vi "GET_Issues.vi"(6 "progress ref":refnum<vi>, 8 "error in (no error)":errorcluster, 11 "series_class in":refnum<class "series_class.lvclass">) -> (0 "error out":errorcluster, 3 "series_class out":refnum<class "series_class.lvclass">)   [LabVIEW 2024, in "series_class.lvclass"]
uses:
  series_class.lvclass
  series_class.lvclass/series_class.ctl
  issue_class/issue_class.lvclass
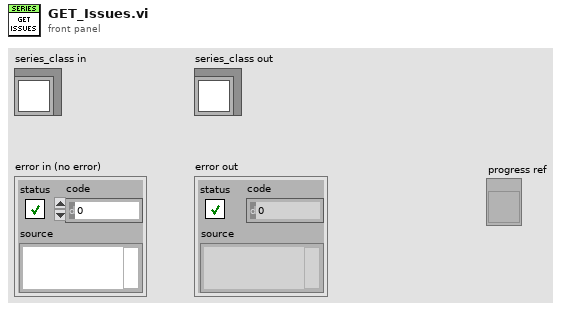
[diagram p1: front panel]
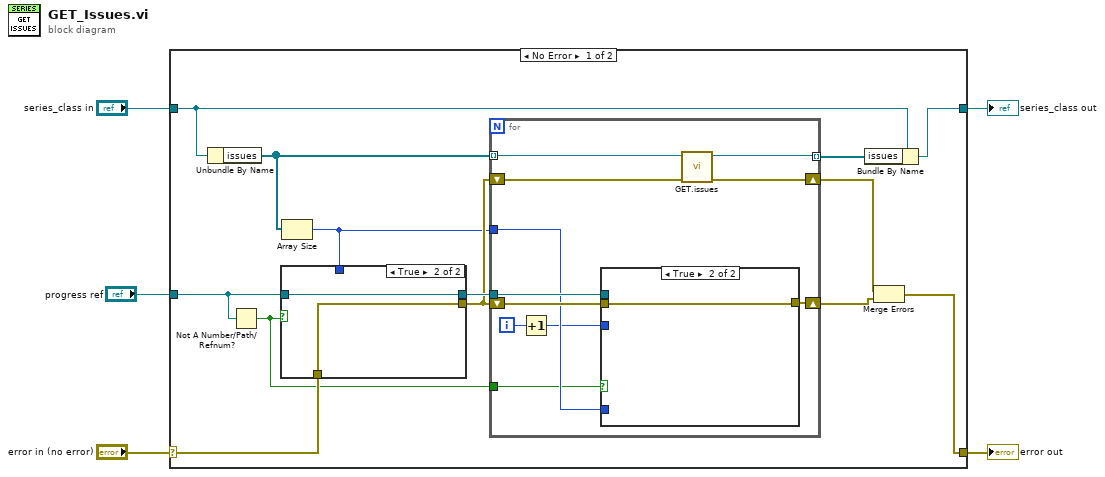
[diagram p0: block diagram]
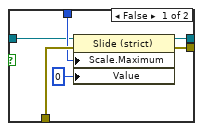
[diagram p2: hidden frame]
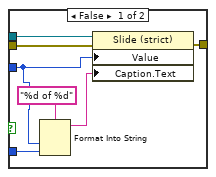
[diagram p3: hidden frame]
diagram:
  n1 = case shown="No Error" "error in (no error)" {
    selector: "error in (no error)" -> [w13 w47]
    tunnel: [w9 w47] -> w4
    tunnel: [w17 w46] -> w2
    tunnel: "series_class in" -> [w18 w46]
    tunnel: "progress ref" -> [w7 _]
    frame No Error {
      n2 = Unbundle By Name(w18) -> ("issues"=w14:refnum<class "issue_class.lvclass">[])
      n3 = Not A Number/Path/Refnum?(number/path/refnum=w7) -> (NaN/Path/Refnum?=w6:bool)
      n4 = Array Size(array=w14) -> (size(s)=w8:i32)
      n5 = case shown="True" w6 {
        tunnel: [w23 w26] -> w15
        tunnel: w13 -> [w22 w25]
        tunnel: [w21 w25] -> w12
        tunnel: w8 -> [w20 _]
        tunnel: w7 -> [w19 w26]
        frame False {
          n6 = property class="Slide (strict)"(reference=w19, error in=w22, "Scale.Maximum"=w20, "Value"=0) -> (reference out=w23:refnum<vi>, error out=w21:errorcluster)
        }
        frame True {
        }
      }
      n7 = for {
        tunnel: w14 -> [w37] mode=indexing
        tunnel: [w36] -> w16 mode=indexing
        shift-right: [w34] -> w11
        shift-left: w12 -> [w35]
        tunnel: w15 -> [w33]
        shift-right: [w30] -> w10
        shift-left: w12 -> [w31]
        tunnel: w8 -> [w29]
        tunnel: w6 -> [w27]
        i -> [w32]
        n8 = Increment(x=w32) -> (x+1=w28:i32)
        n9 = case shown="True" w27 {
          tunnel: w33 -> [w44 _]
          tunnel: w31 -> [w43 w45]
          tunnel: [w42 w45] -> w30
          tunnel: w29 -> [w40 _]
          tunnel: w28 -> [w39 _]
          frame False {
            n10 = Format Into String(format string="%d of %d", w39, w40) -> (resulting string=w38:string)  [unwired: 2 in, 1 out]
            n11 = property class="Slide (strict)"(reference=w44, error in=w43, "Value"=w39, "Caption.Text"=w38) -> (error out=w42:errorcluster)  [unwired: 1 out]
          }
          frame True {
          }
        }
        n12 = call "GET.issues.vi"("error in (no error)"=w35, "issue_class in"=w37) -> ("error out"=w34:errorcluster, "issue_class out"=w36:refnum<class "issue_class.lvclass">)  [unwired: 8 in]
      }
      n13 = Bundle By Name(cluster=w18, "issues"=w16) -> (w17:refnum<class "series_class.lvclass">)
      n14 = Merge Errors(w11, w10) -> (w9:errorcluster)
    }
    frame Error {
    }
  }
  "error out" <- w4
  "series_class out" <- w2
